vi "生成测试说明界面.vi"(1 "错误输入（无错误）":errorcluster, 2 "测试说明界面参数":T1) -> (0 "错误输出":errorcluster)   [LabVIEW 2015]
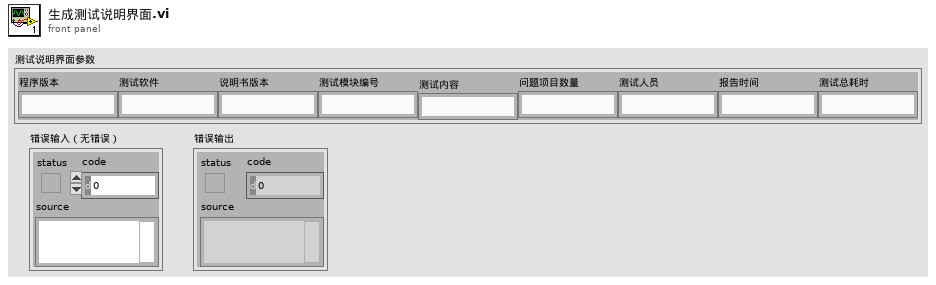
[diagram p1: front panel]
types:
  T1 = typedef "测试说明界面参数.ctl" = cluster{"程序版本":string, "测试软件":string, "说明书版本":string, "测试模块编号":string, "测试内容":string, "问题项目数量":string, "测试人员":string, "报告时间":string, "测试总耗时":string}
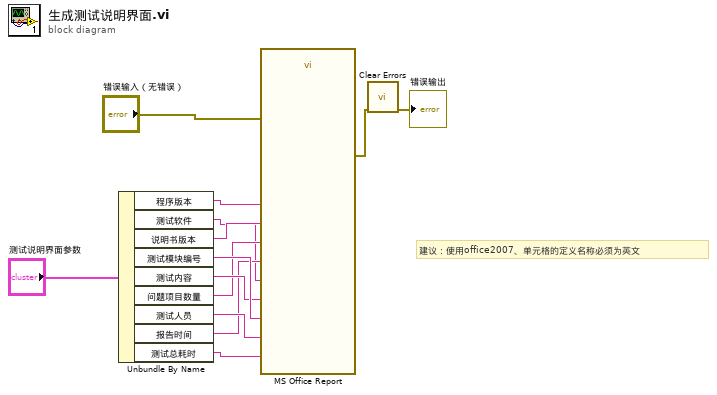
[diagram p0: block diagram]
diagram:
  # "建议：使用office2007、单元格的定义名称必须为英文"
  n1 = Unbundle By Name("测试说明界面参数") -> ("程序版本"=w1:string, "测试软件"=w2:string, "说明书版本"=w9:string, "测试模块编号"=w8:string, "测试内容"=w7:string, "问题项目数量"=w6:string, "测试人员"=w5:string, "报告时间"=w4:string, "测试总耗时"=w3:string)
  n2 = call "MS Office Report"("GPRS_version"=w1, "notebook_vesion"=w9, "number_of_problem"=w6, "production_time"=w4, "software_version"=w2, "error in (no error)"="错误输入（无错误）", "test_content"=w7, "test_ID"=w8, "test_user"=w5, "use_times"=w3) -> ("error out"=w11:errorcluster)  [unwired: 16 in, 1 out]
  n3 = call <vilib>:"Clear Errors.vi"("error in (no error)"=w11) -> ("error out"=→"错误输出":errorcluster)  [unwired: 5 in, 1 out]
